vi "Send MessageRecieved.vi"(7 "Message Priority (Normal)":T2=enum."Normal", 8 "error in (no error)":errorcluster, 10 "clientMessage":T1, 11 "Message Enqueuer":refnum<class "Message Enqueuer.lvclass">) -> (0 "error out":errorcluster, 3 "Message Enqueuer out":refnum<class "Message Enqueuer.lvclass">)   [LabVIEW 2023, in "TCP_Server_Connection_Handler.lvlib" / "MessageRecieved Msg.lvclass"]
doc: "This VI sends the message to an actor."
uses:
  MessageRecieved Msg.lvclass
  <vilib>/ActorFramework/Message Enqueuer/Message Enqueuer.lvclass
  <vilib>/ActorFramework/Message Enqueuer/Message Priority.ctl
  TypeDefinitions/ClientMessage.ctl
  MessageRecieved Msg.lvclass/MessageRecieved Msg.ctl
  <vilib>/ActorFramework/Message Enqueuer/Message Enqueuer.lvclass/Message Enqueuer.ctl
  <vilib>/ActorFramework/Message Priority Queue/Priority Enqueue.vi
  TCP_Server_Connection_Handler.lvlib
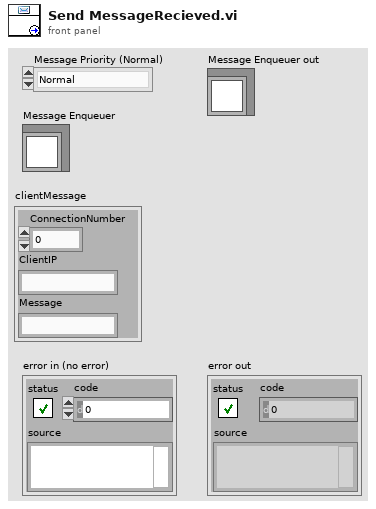
[diagram p1: front panel]
types:
  T1 = typedef "TCP_Server_Connection_Handler.lvlib/ClientMessage.ctl" = cluster{"ConnectionNumber":i32, "ClientIP":string, "Message":string}
  T2 = typedef "Actor Framework.lvlib/Message Enqueuer.lvclass/Message Priority.ctl" = enum16{"Low", "Normal", "High"}
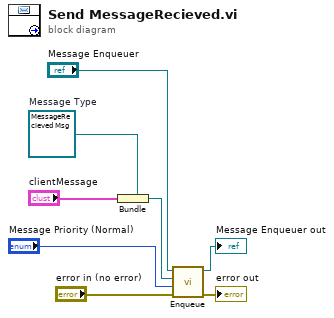
[diagram p0: block diagram]
diagram:
  w5 = refnum<class "MessageRecieved Msg.lvclass"> refnum  # Message Type
  n1 = Bundle(cluster=w5, "clientMessage") -> (w4:refnum<class "MessageRecieved Msg.lvclass">)
  n2 = call <vilib>:"Enqueue.vi"("error in (no error)"="error in (no error)", "Message Priority (Normal)"="Message Priority (Normal)", "Message"=w4, "Message Enqueuer in"="Message Enqueuer") -> ("error out"=→"error out":errorcluster, "Message Enqueuer out"=→"Message Enqueuer out":refnum<class "Message Enqueuer.lvclass">)  [unwired: 6 in]
